vi "ProgramSceme.vi"   [LabVIEW 2011]
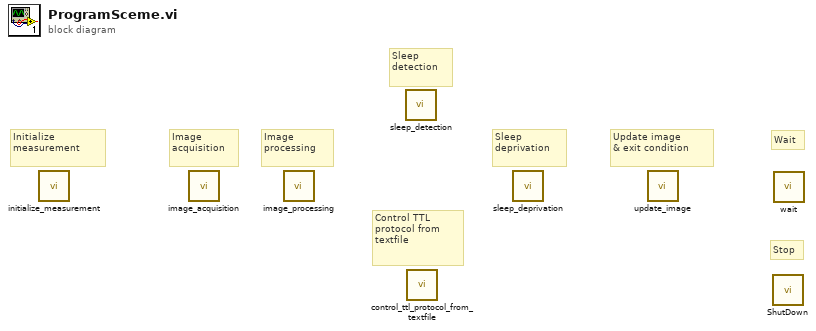
[diagram p0: block diagram]
diagram:
  # "Stop"
  # "Wait"
  # "Update image\n& exit condition"
  # "Sleep \ndeprivation"
  # "Control TTL\nprotocol from\ntextfile"
  # "Sleep\ndetection"
  # "Initialize\nmeasurement"
  # "Image\nacquisition"
  # "Image\nprocessing"
  n1 = call "initialize_measurement.vi"() -> ()  [unwired: 10 in, 1 out]
  n2 = call "image_acquisition.vi"() -> ()  [unwired: 9 in, 3 out]
  n3 = call "image_processing.vi"() -> ()  [unwired: 11 in, 1 out]
  n4 = call "sleep_detection.vi"() -> ()  [unwired: 10 in, 1 out]
  n5 = call "control_ttl_protocol_from_textfile.vi"() -> ()  [unwired: 11 in, 1 out]
  n6 = call "sleep_deprivation.vi"() -> ()  [unwired: 6 in, 1 out]
  n7 = call "update_image.vi"() -> ()  [unwired: 10 in, 2 out]
  n8 = call <userlib>:"ShutDown.vi"() -> ()  [unwired: 2 in, 2 out]
  n9 = call "wait.vi"() -> ()  [unwired: 10 in, 2 out]
